vi "Configure Trigger Model Source Output Block.vi"(8 "error in (no error)":errorcluster, 9 "Output State (OFF)":bool, 10 "Block Number (1)":i32=1 min=1 format="%#.6g", 11 "VISA resource name":refnum<visa-resource-name>) -> (0 "error out":errorcluster, 3 "VISA resource name out":refnum<visa-resource-name>)   [LabVIEW 2022 SP3, in "Keithley 2450.lvlib"]
doc: "This VI defines a trigger block that turns the output source on or off."
uses:
  Keithley 2450.lvlib
panel:
  # "ON"
  # "OFF"
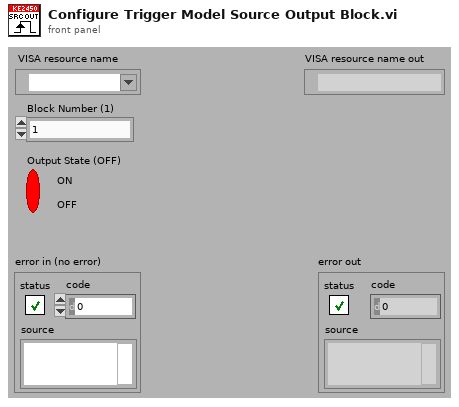
[diagram p1: front panel]
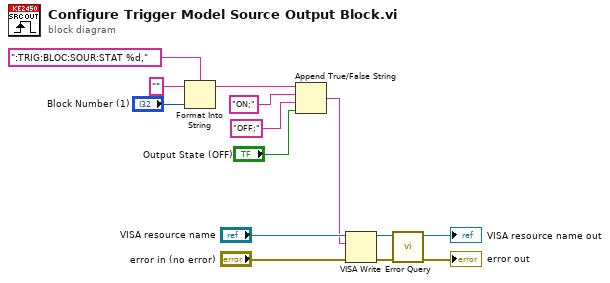
[diagram p0: block diagram]
diagram:
  n1 = Format Into String(format string=":TRIG:BLOC:SOUR:STAT %d,", initial string="", "Block Number (1)") -> (resulting string=w3:string)  [unwired: 1 in, 1 out]
  n2 = Append True/False String(1:"Output State (OFF)", 2:"OFF;" ("false string"), 3:"ON;" ("true string"), 4:w3) -> (0:w5:string)
  n3 = VISA Write(VISA resource name="VISA resource name", write buffer=w5, error in (no error)="error in (no error)") -> (VISA resource name out=w10:refnum<visa-resource-name>, error out=w9:errorcluster)  [unwired: 1 out]
  n4 = call "Error Query.vi"("error in (no error)"=w9, "VISA resource name"=w10) -> ("error out"=→"error out":errorcluster, "VISA resource name out"=→"VISA resource name out":refnum<visa-resource-name>)  [unwired: 8 out]
